vi "TL_initialize_Z_ramp.vi"(0 "queue piezo":refnum<queue>, 1 "Exp time (s)":sgl=0.05 format="%#_3g", 2 "# cycle":i32, 5 "TL array":dbl[][](array[numeric]), 7 "queue DAQ":refnum<queue>, 9 "# channel":i32, 11 "error in":errorcluster, 12 "queue ASI stage":refnum<queue>) -> (3 "Ramp":dbl[](array[numeric]), 4 "# steps":i32, 10 "BF?":bool, 15 "error out":errorcluster)   [LabVIEW 2015]
uses:
  CONTROLS/Q_MCL_piezo_element.ctl
  CONTROLS/Q_DAQ_element.ctl
  CONTROLS/Q_ASI_stage_element.ctl
  GLOBAL/Global_MCL_piezo.vi
  GLOBAL/Global_DAQ.vi
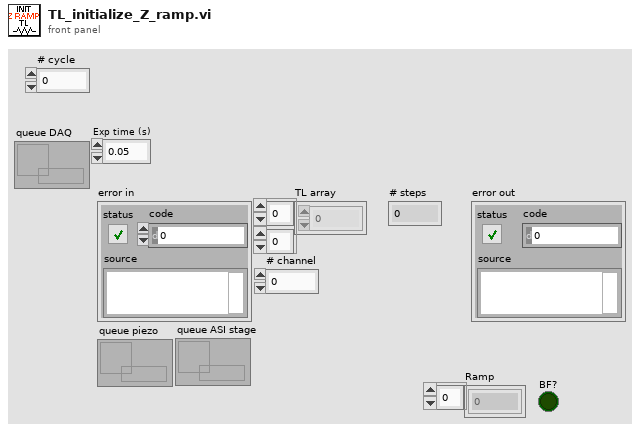
[diagram p1: front panel]
types:
  T1 = typedef "Q_MCL_piezo_element.ctl" = cluster{"variant":variant, "Instruction":enum16{"Piezo_idle", "Piezo_initialize", "Piezo_error", "Piezo_security_stop", "Piezo_read_z", "Piezo_move_z", "Piezo_keyboard_move", "Piezo_close_autofocus_calibration_ramp", "Piezo_change_init_state", "Piezo_init_autofocus", "Piezo_init_autofocus_merFISH_TL", "Piezo_autofocus", "Piezo_autofocus_merFISH_TL", "Piezo_stop_autofocus", "Piezo_stop_autofocus_merFISH_TL", "Piezo_autofocus_lost", "Piezo_resume_autofocus_merFISH_TL", "Piezo_check_z_position_merFISH_TL", "Piezo_init_ramp", "Piezo_move_z_ramp", "Piezo_close_ramp", "Piezo_close_merFISH", "Piezo_init_TL", "Piezo_close_ramp_TL", "Piezo_close_TL", "Piezo_stop"}}
  T2 = typedef "Q_DAQ_element.ctl" = cluster{"variant":variant, "Instruction":enum16{"DAQ_idle", "DAQ_initialize", "DAQ_error", "DAQ_security_stop", "DAQ_start_QPD", "DAQ_change_QPD_display", "DAQ_read_display_QPD_signal", "DAQ_QPD_init_autofocus", "DAQ_read_display_send_QPD_signal", "DAQ_close_autofocus_calibration_ramp", "DAQ_close_autofocus", "DAQ_405", "DAQ_488", "DAQ_561", "DAQ_641", "DAQ_zero_all", "DAQ_init_single_scan", "DAQ_single_scan", "DAQ_two_way_valve", "DAQ_init_merFISH", "DAQ_scan_merFISH", "DAQ_photobleaching_merFISH", "DAQ_close_merFISH", "DAQ_init_TL", "DAQ_synchro_TL", "DAQ_close_task_TL", "DAQ_close_TL", "DAQ_stop"}}
  T3 = typedef "Q_ASI_stage_element.ctl" = cluster{"variant":variant, "Instruction":enum16{"ASI_idle", "ASI_initialize", "ASI_error", "ASI_security_stop", "ASI_read_XYZ", "ASI_up", "ASI_down", "ASI_left", "ASI_right", "ASI_save_XY", "ASI_move_to_XY", "ASI_brightfield", "ASI_init_scan", "ASI_init_merFISH", "ASI_move_to_XY_merFISH", "ASI_move_to_Z_merFISH", "ASI_init_autofocus_search_merFISH", "ASI_close_autofocus_search_merFISH", "ASI_adjust_piezo_autofocus_merFISH", "ASI_set_piezo_autofocus_to_reference_position_merFISH_TL", "ASI_close_merFISH", "ASI_init_TL", "ASI_move_mosaic_TL", "ASI_brightfield_TL", "ASI_close_TL", "ASI_stop"}}
  T4 = enum16{"DAQ_idle", "DAQ_initialize", "DAQ_error", "DAQ_security_stop", "DAQ_start_QPD", "DAQ_change_QPD_display", "DAQ_read_display_QPD_signal", "DAQ_QPD_init_autofocus", "DAQ_read_display_send_QPD_signal", "DAQ_close_autofocus_calibration_ramp", "DAQ_close_autofocus", "DAQ_405", "DAQ_488", "DAQ_561", "DAQ_641", "DAQ_zero_all", "DAQ_init_single_scan", "DAQ_single_scan", "DAQ_two_way_valve", "DAQ_init_merFISH", "DAQ_scan_merFISH", "DAQ_photobleaching_merFISH", "DAQ_close_merFISH", "DAQ_init_TL", "DAQ_synchro_TL", "DAQ_close_task_TL", "DAQ_close_TL", "DAQ_stop"}
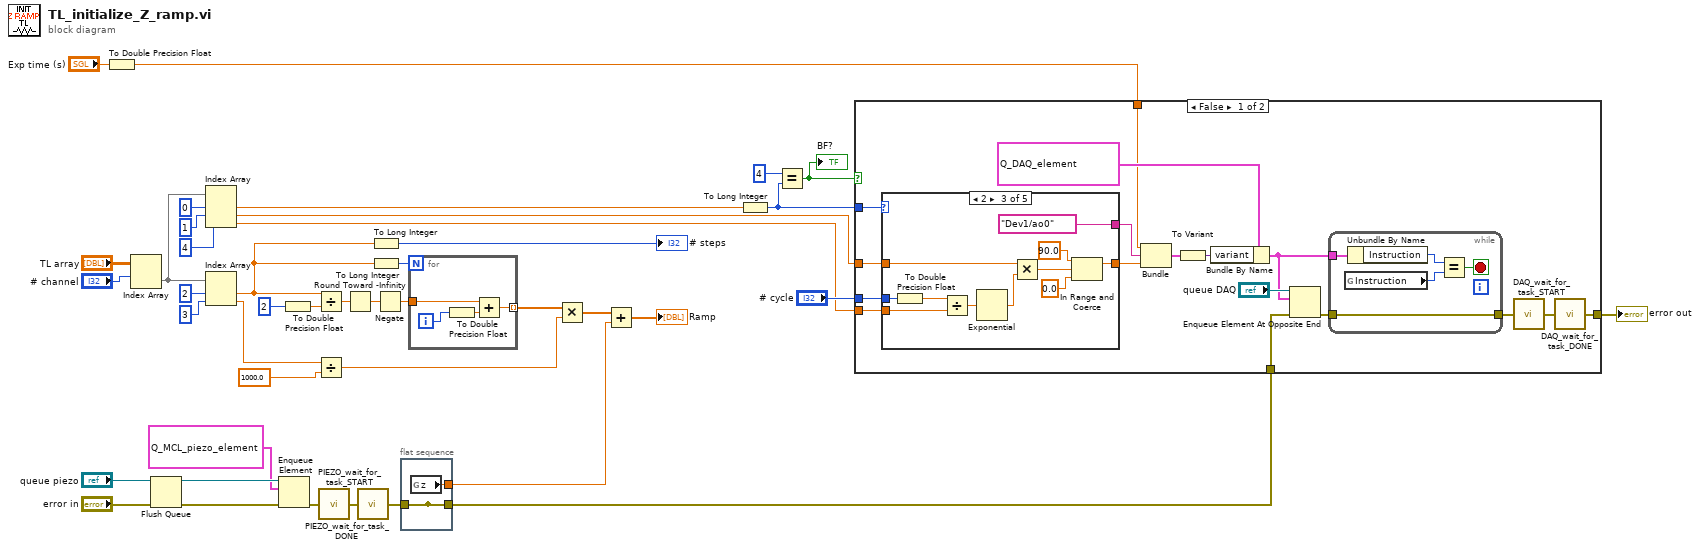
[diagram p0: block diagram]
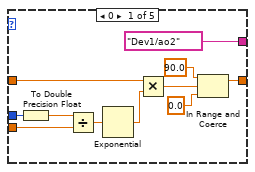
[diagram p2: hidden frame]
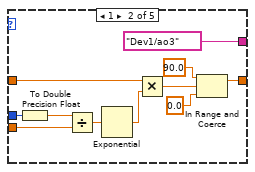
[diagram p3: hidden frame]
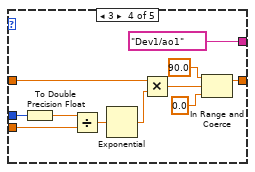
[diagram p4: hidden frame]
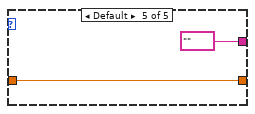
[diagram p5: hidden frame]
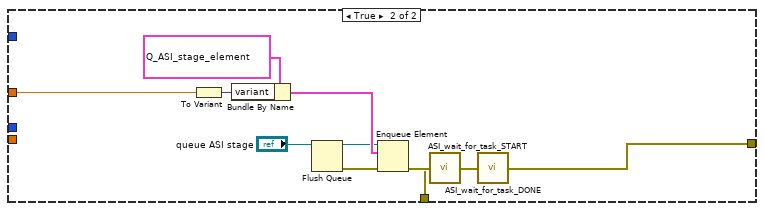
[diagram p6: hidden frame]
diagram:
  n1 = To Double Precision Float(number="Exp time (s)") -> (double precision float=w10:dbl)
  n2 = Index Array(array="TL array", index (row)="# channel") -> (element=w7:dbl[])  [unwired: 1 in]
  n3 = Flush Queue(queue="queue piezo", error in (no error)="error in") -> (queue out=w24:refnum<queue>, error out=w23:errorcluster)  [unwired: 1 out]
  n4 = Index Array(array=w7, index #1=0 ("index"), index #2=1 ("index"), index #3=4 ("index")) -> (element #1=w3:dbl, element #2=w2:dbl, element #3=w1:dbl)
  n5 = Index Array(array=w7, index #1=2 ("index"), index #2=3 ("index")) -> (element #1=w30:dbl, element #2=w29:dbl)
  n6 = Enqueue Element(queue=w24, element=T1 {"variant"=variant, "Instruction"=enum."Piezo_init_ramp"} ("Q_MCL_Piezo"), error in (no error)=w23) -> (error out=w26:errorcluster)  [unwired: 1 in, 2 out]
  n7 = To Double Precision Float(number=2 ("y")) -> (double precision float=w41:dbl)
  n8 = Divide(x=w30, y=w41) -> (x/y=w40:dbl)
  n9 = Divide(x=w29, y=1000.0) -> (x/y=w35:dbl)
  n10 = call "PIEZO_wait_for_task_START.vi"("error in"=w26) -> ("error out"=w25:errorcluster)
  n11 = Round Toward -Infinity(1:w40) -> (0:w39:dbl)
  n12 = call "PIEZO_wait_for_task_DONE.vi"("error in"=w25) -> ("error out"=w27:errorcluster)
  n13 = To Long Integer(number=w30) -> (32bit integer=→"# steps":i32)
  n14 = To Long Integer(number=w30) -> (32bit integer=w28:i32)
  n15 = Negate(x=w39) -> (-x=w38:dbl)
  n16 = flat-sequence {
    tunnel: w27 -> [w43]
    tunnel: [w43] -> _
    tunnel: [w44] -> w18
    tunnel: [w43] -> w15
    frame #0 {
      n17 = global read "Global_MCL_piezo.vi" "z"() -> (w44:dbl)
    }
  }
  n18 = for {
    N: w28 -> [_]
    tunnel: w38 -> [w48]
    tunnel: [w45] -> w36 mode=indexing
    i -> [w47]
    n19 = To Double Precision Float(number=w47) -> (double precision float=w46:dbl)
    n20 = Add(x=w48, y=w46) -> (x+y=w45:dbl)
  }
  n21 = Multiply(x=w36, y=w35) -> (x*y=w19:dbl[])
  n22 = Add(x=w19, y=w18) -> (x+y=→"Ramp":dbl[])
  n23 = To Long Integer(number=w3) -> (32bit integer=w14:i32)
  n24 = Equal?(x=4, y=w14) -> (x = y?=w12:bool)
  "BF?" <- w12
  n25 = case shown="False" w12 {
    tunnel: w2 -> [w55 w125]
    tunnel: w15 -> [w60 w117]
    tunnel: w14 -> [w58 _]
    tunnel: w10 -> [w57 _]
    tunnel: [w56 w121] -> w9
    tunnel: "# cycle" -> [w53 _]
    tunnel: w1 -> [w52 _]
    frame False {
      n26 = case shown="2" w58 {
        tunnel: [tag "Dev1/ao2" ("Analogic input") tag "Dev1/ao3" ("Analogic input") tag "Dev1/ao0" ("Analogic input") tag "Dev1/ao1" ("Analogic input") tag "" ("Analogic input")] -> w61
        tunnel: w55 -> [w77 w88 w99 w110 w115]
        tunnel: [w75 w86 w97 w108 w115] -> w54
        tunnel: w53 -> [w80 w91 w102 w113 _]
        tunnel: w52 -> [w71 w82 w93 w104 _]
        frame 0 {
          n27 = To Double Precision Float(number=w80) -> (double precision float=w72:dbl)
          n28 = Divide(x=w72, y=w71) -> (x/y=w79:dbl)
          n29 = Exponential(1:w79) -> (0:w78:dbl)
          n30 = Multiply(x=w77, y=w78) -> (x*y=w76:dbl)
          n31 = In Range and Coerce(upper limit=90.0, x=w76, lower limit=0.0) -> (coerced(x)=w75:dbl)  [unwired: 1 out]
        }
        frame 1 {
          n32 = To Double Precision Float(number=w91) -> (double precision float=w83:dbl)
          n33 = Divide(x=w83, y=w82) -> (x/y=w90:dbl)
          n34 = Exponential(1:w90) -> (0:w89:dbl)
          n35 = Multiply(x=w88, y=w89) -> (x*y=w87:dbl)
          n36 = In Range and Coerce(upper limit=90.0, x=w87, lower limit=0.0) -> (coerced(x)=w86:dbl)  [unwired: 1 out]
        }
        frame 2 {
          n37 = To Double Precision Float(number=w102) -> (double precision float=w94:dbl)
          n38 = Divide(x=w94, y=w93) -> (x/y=w101:dbl)
          n39 = Exponential(1:w101) -> (0:w100:dbl)
          n40 = Multiply(x=w99, y=w100) -> (x*y=w98:dbl)
          n41 = In Range and Coerce(upper limit=90.0, x=w98, lower limit=0.0) -> (coerced(x)=w97:dbl)  [unwired: 1 out]
        }
        frame 3 {
          n42 = To Double Precision Float(number=w113) -> (double precision float=w105:dbl)
          n43 = Divide(x=w105, y=w104) -> (x/y=w112:dbl)
          n44 = Exponential(1:w112) -> (0:w111:dbl)
          n45 = Multiply(x=w110, y=w111) -> (x*y=w109:dbl)
          n46 = In Range and Coerce(upper limit=90.0, x=w109, lower limit=0.0) -> (coerced(x)=w108:dbl)  [unwired: 1 out]
        }
        frame Default {
        }
      }
      n47 = Bundle(w57, "Analogic input"=w61, "BF"=w54) -> (w63:cluster{dbl, "Analogic input":tag, "BF ":dbl})  [unwired: 1 in]
      n48 = To Variant(anything=w63) -> (Variant=w62:variant)
      n49 = Bundle By Name(cluster=T2 {"variant"=variant, "Instruction"=enum."DAQ_synchro_TL"} ("Q_DAQ"), "variant"=w62) -> (w49:T2)
      n50 = Enqueue Element At Opposite End(queue="queue DAQ", element=w49, error in (no error)=w60) -> (error out=w51:errorcluster)  [unwired: 1 in, 2 out]
      n51 = while {
        tunnel: w51 -> [w67]
        tunnel: [w67] -> w50
        tunnel: w49 -> [w66]
        stop <- w69 stop-if-true
        n52 = global read "Global_DAQ.vi" "Instruction"() -> (w70:T4)
        n53 = Unbundle By Name(w66) -> ("Instruction"=w68:T4)
        n54 = Equal?(x=w68, y=w70) -> (x = y?=w69:bool)
      }
      n55 = call "DAQ_wait_for_task_START.vi"("error in"=w50) -> ("error out"=w64:errorcluster)
      n56 = call "DAQ_wait_for_task_DONE.vi"("error in"=w64) -> ("error out"=w56:errorcluster)
    }
    frame True {
      n57 = To Variant(anything=w125) -> (Variant=w126:variant)
      n58 = Bundle By Name(cluster=T3 {"variant"=variant, "Instruction"=enum."ASI_brightfield_TL"} ("element"), "variant"=w126) -> (w124:T3)
      n59 = Flush Queue(queue="queue ASI stage", error in (no error)=w117) -> (queue out=w119:refnum<queue>, error out=w118:errorcluster)  [unwired: 1 out]
      n60 = Enqueue Element(queue=w119, element=w124, error in (no error)=w118) -> (error out=w123:errorcluster)  [unwired: 1 in, 2 out]
      n61 = call "ASI_wait_for_task_START.vi"("error in"=w123) -> ("error out"=w122:errorcluster)
      n62 = call "ASI_wait_for_task_DONE.vi"("error in"=w122) -> ("error out"=w121:errorcluster)
    }
  }
  "error out" <- w9
